vi "Lian_Reshaping_Array_Data.vi"() -> ()   [LabVIEW 2020]
panel:
  out "Processed Data":string
  in  "Raw Data":dbl[][](array[numeric])=[[1.0, 2.0, 3.0, 4.0, 5.0], [100.0, 101.0, 102.0, 103.0, 104.0], [6.0, 7.0, 8.0, 9.0, 10.0], [105.0, 106.0, 107.0, 108.0, 109.0], [11.0, 12.0, 13.0, 14.0, 15.0], [110.0, 111.0, 112.0, 113.0, 114.0]]
  in  "Raw Data":dbl[][](array[numeric])=[[1.0, 2.0, 3.0, 4.0, 5.0], [100.0, 101.0, 102.0, 103.0, 104.0], [6.0, 7.0, 8.0, 9.0, 10.0], [105.0, 106.0, 107.0, 108.0, 109.0], [11.0, 12.0, 13.0, 14.0, 15.0], [110.0, 111.0, 112.0, 113.0, 114.0]]
  in  "file path (use dialog)":path=path "C:/Users/Billy/Desktop/DAQ/HW/HW 5/Reshaping_Array_Data_Lian.txt"
  in  "Raw Data":dbl[][](array[numeric])=[[1.0, 2.0, 3.0, 4.0, 5.0], [100.0, 101.0, 102.0, 103.0, 104.0], [6.0, 7.0, 8.0, 9.0, 10.0], [105.0, 106.0, 107.0, 108.0, 109.0], [11.0, 12.0, 13.0, 14.0, 15.0], [110.0, 111.0, 112.0, 113.0, 114.0]]
  # "Reshaping Array Data"
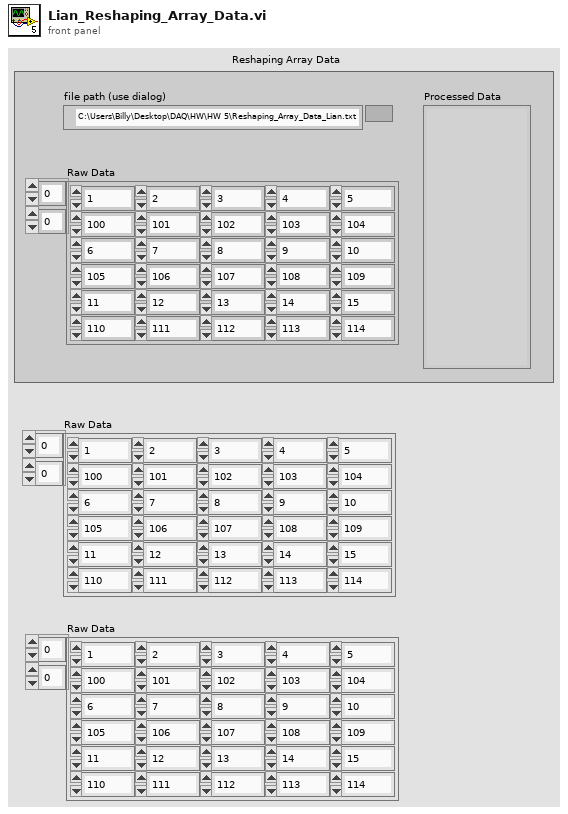
[diagram p1: front panel]
types:
  T1 = enum16{"open", "replace", "create", "open or create", "replace or create", "replace or create with confirmation"}
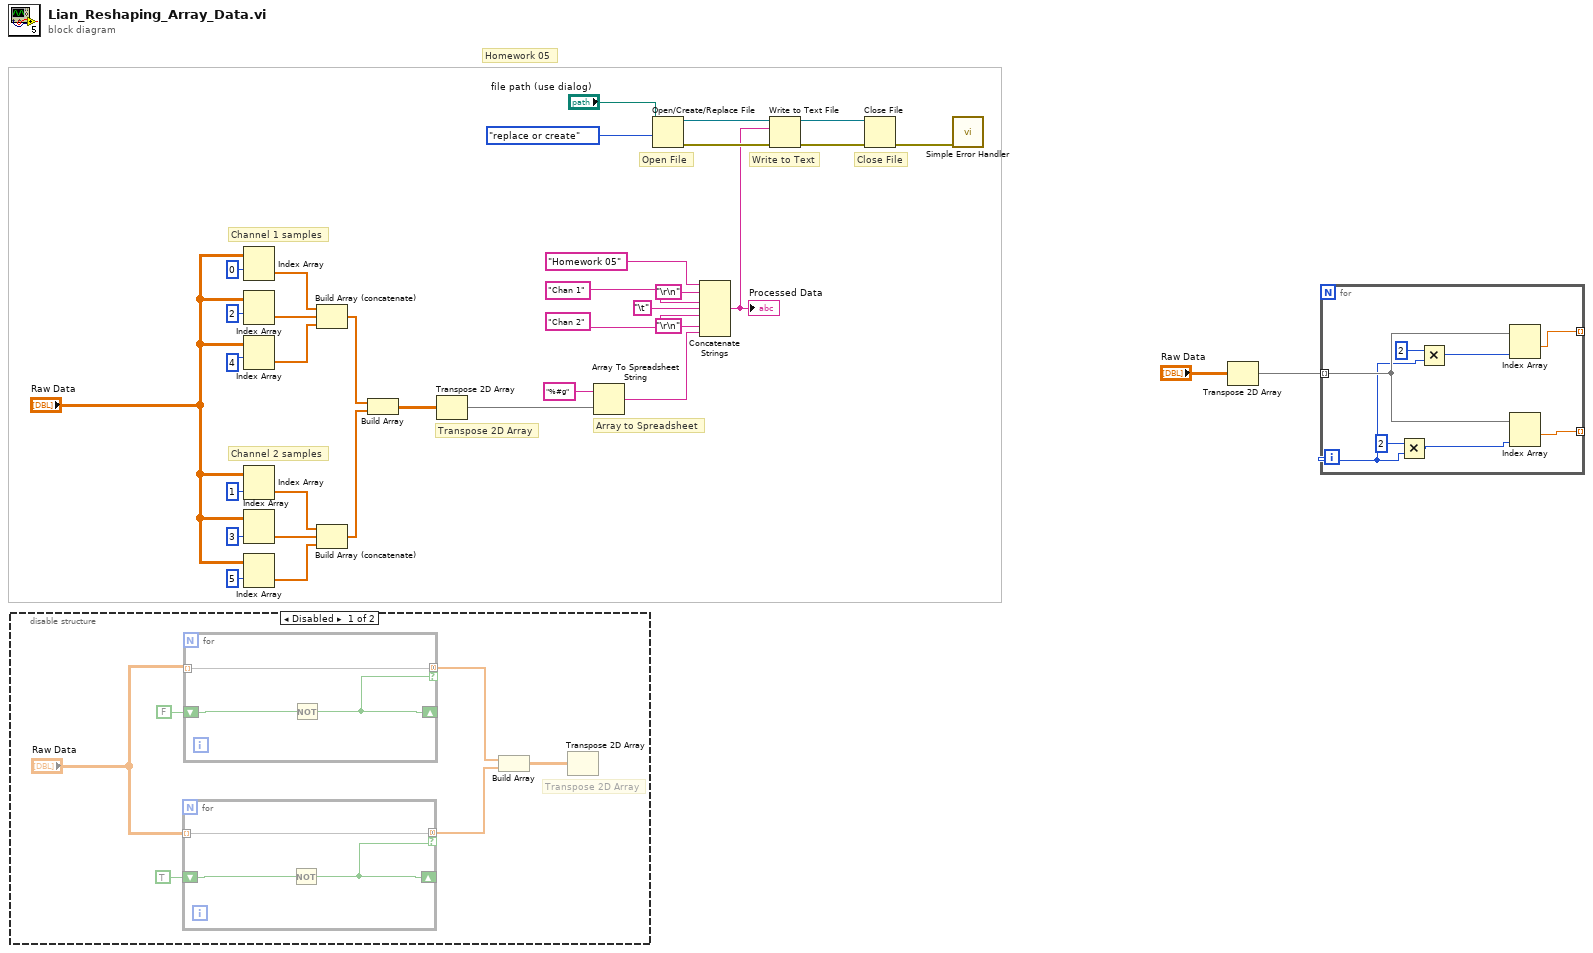
[diagram p0: block diagram]
diagram:
  # "Homework 05"
  # "Transpose 2D Array"
  # "Array to Spreadsheet"
  # "Write to Text"
  # "Close File"
  # "Open File"
  # "Channel 2 samples"
  # "Channel 1 samples"
  n1 = disable-structure shown="Disabled" {
    frame Disabled {
      # "Transpose 2D Array"
      n2 = for {
        shift-right: [w43] -> _
        shift-left: TRUE -> [w44]
        tunnel: [w42] -> w38 mode=concatenating if=w43
        tunnel: "Raw Data" -> [w42] mode=indexing
        n3 = Not(x=w44) -> (.not. x?=w43:bool)
      }
      n4 = for {
        shift-right: [w46] -> _
        shift-left: FALSE -> [w47]
        tunnel: [w45] -> w39 mode=concatenating if=w46
        tunnel: "Raw Data" -> [w45] mode=indexing
        n5 = Not(x=w47) -> (.not. x?=w46:bool)
      }
      n6 = Build Array(w39, w38) -> (w36:dbl[][])
      n7 = Transpose 2D Array(2D array=w36) -> ()  [unwired: 1 out]
    }
    frame Enabled {
    }
  }
  n8 = Index Array(array="Raw Data", index (row)=0) -> (element=w20:dbl[])  [unwired: 1 in]
  n9 = Index Array(array="Raw Data", index (row)=2) -> (element=w31:dbl[])  [unwired: 1 in]
  n10 = Index Array(array="Raw Data", index (row)=4) -> (element=w21:dbl[])  [unwired: 1 in]
  n11 = Index Array(array="Raw Data", index (row)=1) -> (element=w26:dbl[])  [unwired: 1 in]
  n12 = Index Array(array="Raw Data", index (row)=3) -> (element=w27:dbl[])  [unwired: 1 in]
  n13 = Index Array(array="Raw Data", index (row)=5) -> (element=w25:dbl[])  [unwired: 1 in]
  n14 = Build Array (concatenate)(w20, w31, w21) -> (w24:dbl[])
  n15 = Build Array (concatenate)(w26, w27, w25) -> (w23:dbl[])
  n16 = Build Array(w24, w23) -> (w22:dbl[][])
  n17 = Transpose 2D Array(2D array=w22) -> (transposed array=w16:dbl[][])
  n18 = Array To Spreadsheet String(array=w16, 3:"%#g" ("format string")) -> (spreadsheet string=w6:string)  [unwired: 1 in]
  n19 = Open/Create/Replace File(file path (use dialog)="file path (use dialog)", operation (0:open)=T1."replace or create") -> (refnum out=w11:refnum<file>, error out=w12:errorcluster)  [unwired: 4 in, 1 out]
  n20 = Concatenate Strings("Homework 05", "\r\n", "Chan 1", "\t", "Chan 2", "\r\n", w6) -> (w10:string)
  "Processed Data" <- w10
  n21 = Write to Text File(file (use dialog)=w11, text=w10, error in=w12) -> (refnum out=w15:refnum<file>, error out=w14:errorcluster)  [unwired: 1 in, 1 out]
  n22 = Close File(refnum=w15, error in=w14) -> (error out=w13:errorcluster)  [unwired: 1 out]
  n23 = call <vilib>:"Simple Error Handler.vi"("error in (no error)"=w13) -> ()  [unwired: 4 in, 5 out]
  n24 = Transpose 2D Array(2D array="Raw Data") -> (transposed array=w2:dbl[][])
  n25 = for {
    tunnel: w2 -> [w55] mode=indexing
    tunnel: [w54] -> _ mode=indexing
    tunnel: [w53] -> _ mode=indexing
    i -> [w51]
    n26 = Multiply(x=2, y=w51) -> (x*y=w49:i32)
    n27 = Multiply(x=2, y=w51) -> (x*y=w48:i32)
    n28 = Index Array(array=w55, index #2=w48) -> (element #1=w54:dbl)  [unwired: 1 in, 1 out]
    n29 = Index Array(array=w55, index #2=w49) -> (element #1=w53:dbl)  [unwired: 1 in, 1 out]
  }
